vi "PythonName.vi"(6 "add self":bool=TRUE, 8 "error in":errorcluster, 11 "Pane in":refnum<class "Pane.lvclass">) -> (0 "error out":errorcluster, 3 "Pane out":refnum<class "Pane.lvclass">, 5 "name":string, 7 "UID":string)   [LabVIEW 2014, in "Pane.lvclass"]
uses:
  Pane.lvclass
  Python/Parsing/Python Functions.lvlib
  GObject/GObject.lvclass
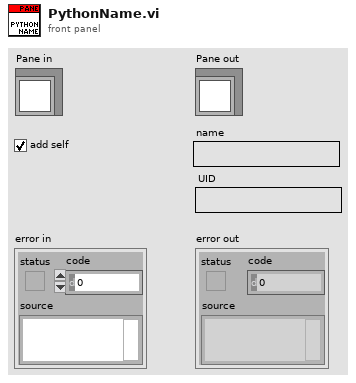
[diagram p1: front panel]
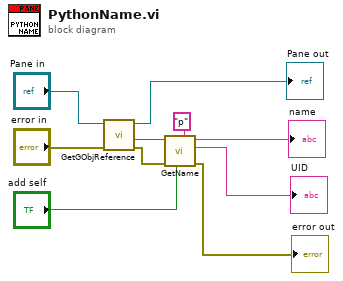
[diagram p0: block diagram]
diagram:
  n1 = call "GetGObjReference.vi"("error in"="error in", "GObject in"="Pane in") -> ("error out"=w9:errorcluster, "reference out"=w10:refnum<vi>, "GObject out"=→"Pane out":refnum<class "Pane.lvclass">)  [unwired: 5 in]
  n2 = call "GetName.vi"("base name"="p", "add self"="add self", "error in"=w9, "GObj Refnum"=w10) -> ("error out"=→"error out":errorcluster, "UID"=→"UID":string, "name"=→"name":string)  [unwired: 5 in]
